vi "gh-cli Release Create.vi"(8 "error in (no error)":errorcluster, 10 "Options":string, 11 "Git in":refnum<class "Git.lvclass">) -> (0 "error out":errorcluster, 2 "standard output":string, 3 "Git out":refnum<class "Git.lvclass">)   [LabVIEW 2019, in "Git.lvclass"]
doc: "gh release create [<b>Options</b>]: Create a new GitHub Release for a repository.\n\nA list of asset files may be given to upload to the new release. To define a display label for an asset, append text starting with # after the file name.\n\nIf a matching git tag does not yet exist, one will automatically get created from the latest state of the default branch. Use --target to override this. To fetch the new tag locally after the release, do git fetch --tags origin.\n\nTo create a release from an annotated git tag, first create one locally with git, push the tag to GitHub, then run this command.\n\nWhen using automatically generated release notes, a release title will also be automatically generated unless a title was explicitly passed. Additional release notes can be prepended to automatically generated notes by using the notes parameter.\n\n<b>Options</b>\n--discussion-category <string>: Start a discussion in the specified category\n-d, --draft: Save the release as a draft instead of publishing it\n--generate-notes: Automatically generate title and notes for the release\n-n, --notes <string>: Release notes\n-F, --notes-file <file>: Read release notes from file (use \"-\" to read from standard input)\n-p, --prerelease: Mark the release as a prerelease\n--target <branch>: Target branch or full commit SHA (default: main branch)\n-t, --title <string>: Release title\n-R, --repo <[HOST/]OWNER/REPO>: Select another repository using the [HOST/]OWNER/REPO format \n\nhttps://cli.github.com/manual"
uses:
  Git.lvclass
  Git.lvclass/Git.ctl
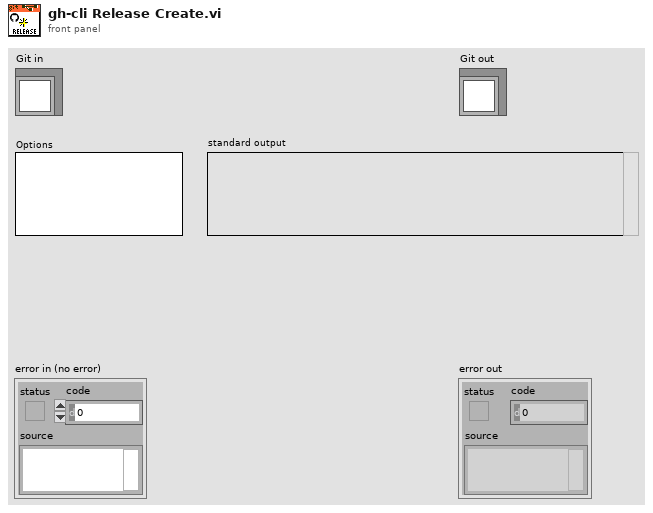
[diagram p1: front panel]
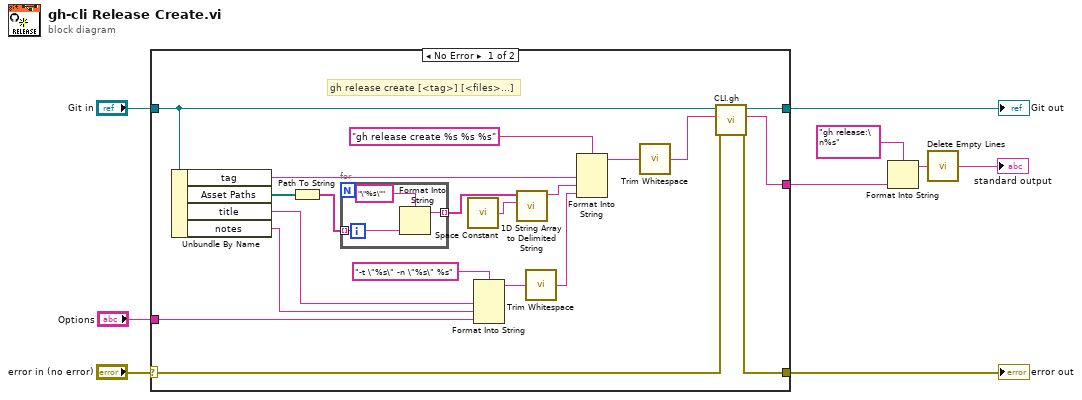
[diagram p0: block diagram]
diagram:
  n1 = case shown="No Error" "error in (no error)" {
    selector: "error in (no error)" -> [w28 w34]
    tunnel: [w27 w34] -> w8
    tunnel: [w29 w33] -> w6
    tunnel: "Git in" -> [w26 w33]
    tunnel: "Options" -> [w23 _]
    tunnel: [w14 _] -> w2
    frame No Error {
      # "gh release create [<tag>] [<files>...]"
      n2 = Unbundle By Name(w26) -> ("tag"=w10:string, "Asset Paths"=w21:path[], "title"=w12:string, "notes"=w13:string)
      n3 = Path To String(path=w21) -> (string=w11:string[])
      n4 = for {
        tunnel: w11 -> [w31] mode=indexing
        tunnel: [w30] -> w15 mode=indexing
        n5 = Format Into String(format string="\"%s\"", w31) -> (resulting string=w30:string)  [unwired: 2 in, 1 out]
      }
      n6 = call <vilib>:"Space Constant.vi"() -> ("String"=w22:string)
      n7 = Format Into String(format string="-t \"%s\" -n \"%s\" %s" ("Options"), w12, w13, w23) -> (resulting string=w20:string)  [unwired: 2 in, 1 out]
      n8 = call <vilib>:"1D String Array to Delimited String.vi"("delimiter"=w22, "string array"=w15) -> ("delimited string"=w16:string)  [unwired: 9 in]
      n9 = call <vilib>:"Trim Whitespace.vi"("string"=w20) -> ("trimmed string"=w19:string)  [unwired: 1 in]
      n10 = Format Into String(format string="gh release create %s %s %s" ("Options"), w10, w16, w19) -> (resulting string=w18:string)  [unwired: 2 in, 1 out]
      n11 = call <vilib>:"Trim Whitespace.vi"("string"=w18) -> ("trimmed string"=w17:string)  [unwired: 1 in]
      n12 = call "CLI.gh.vi"("error in (no error)"=w28, "Command"=w17, "Git in"=w26) -> ("error out"=w27:errorcluster, "standard output"=w14:string, "Git out"=w29:refnum<class "Git.lvclass">)  [unwired: 4 in, 2 out]
    }
    frame Error {
    }
  }
  "error out" <- w8
  "Git out" <- w6
  n13 = Format Into String(format string="gh release:\n%s", w2) -> (resulting string=w3:string)  [unwired: 2 in, 1 out]
  n14 = call "Delete Empty Lines.vi"("String"=w3) -> ("delimited string"=→"standard output":string)
